vi "DSO1K Acquire Waveform.vi"() -> ()   [LabVIEW 2009]
doc: "This example shows how to use autosetup and acquire a waveform on a single channel."
uses:
  <instrlib>/DSO1K/Public/Data/Read Waveform (Single).vi
  <instrlib>/DSO1K/DSO1K.lvlib
panel:
  in  "Timeout (40000 ms)":u32=40000
  in  "Channel (1: Channel 1)":u16(ring)=1 items=["Channel 1"=1, "Channel 2"=2, "Channel 3"=3, "Channel 4"=4]
  out "Waveform Graph":T1(graph)
  in  "VISA resource name":refnum<visa-resource-name>
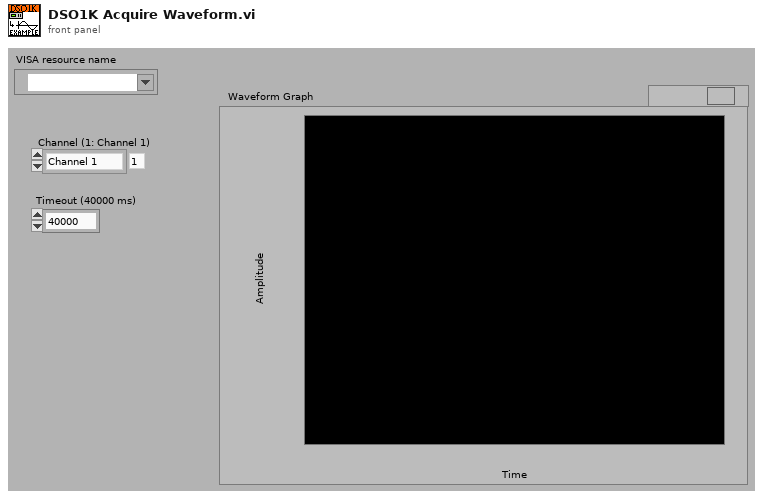
[diagram p1: front panel]
types:
  T1 = cluster{"The start time of the waveform":dbl, dbl, "Waveform":dbl[]}
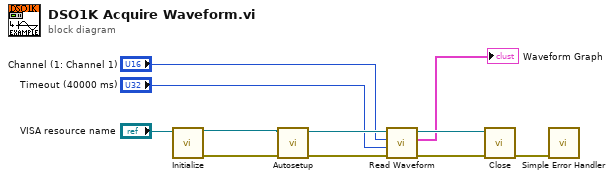
[diagram p0: block diagram]
diagram:
  n1 = call <instrlib>:"Initialize.vi"("VISA resource name"="VISA resource name") -> ("error out"=w7:errorcluster, "VISA resource name out"=w4:refnum<visa-resource-name>)  [unwired: 9 in]
  n2 = call <instrlib>:"Autosetup.vi"("error in (no error)"=w7, "VISA resource name"=w4) -> ("error out"=w6:errorcluster, "VISA resource name out"=w5:refnum<visa-resource-name>)  [unwired: 8 in]
  n3 = call-poly <instrlib>:"Read Waveform.vi"("error in (no error)"=w6, "Timeout (40000 ms)"="Timeout (40000 ms)", "Channel (1: Channel 1)"="Channel (1: Channel 1)", "VISA resource name"=w5) -> ("error out"=w8:errorcluster, "Waveform Graph"=→"Waveform Graph":cluster{dbl, "Sampling Period":dbl, dbl[]}, "VISA resource name out"=w9:refnum<visa-resource-name>)  [unwired: 4 in, 1 out]
  n4 = call <instrlib>:"Close.vi"("error in (no error)"=w8, "VISA resource name"=w9) -> ("error out"=w11:errorcluster)  [unwired: 9 in]
  n5 = call <vilib>:"Simple Error Handler.vi"("error in (no error)"=w11) -> ()  [unwired: 4 in, 5 out]
